vi "MSScript_SubVI_EditorShowTo.vi"(0 "Listbox Ref":refnum<vi>, 1 "Variable In":ext[](array[numeric]), 2 "Variable Index":i32[](array[numeric]), 3 "Variable Name":string, 11 "error in (no error)":errorcluster, 12 "String Color":u32) -> (15 "error out":errorcluster)   [LabVIEW 2018, in "MSScript.lvclass"]
uses:
  MSScript.lvclass
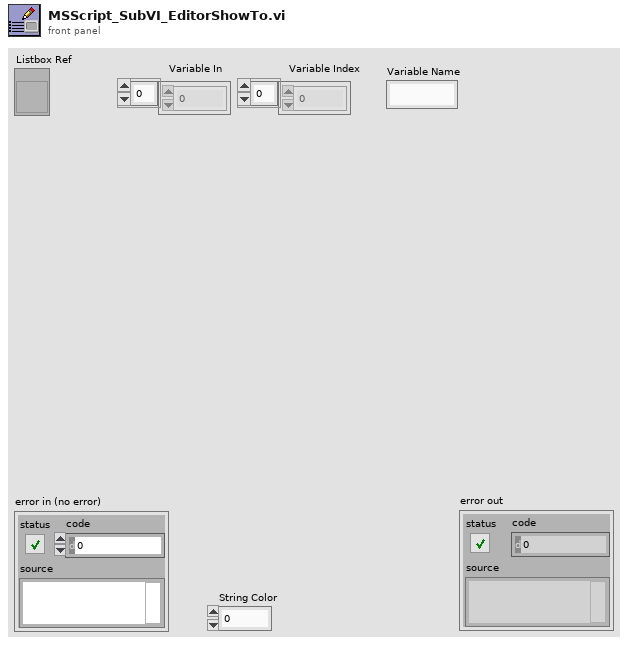
[diagram p1: front panel]
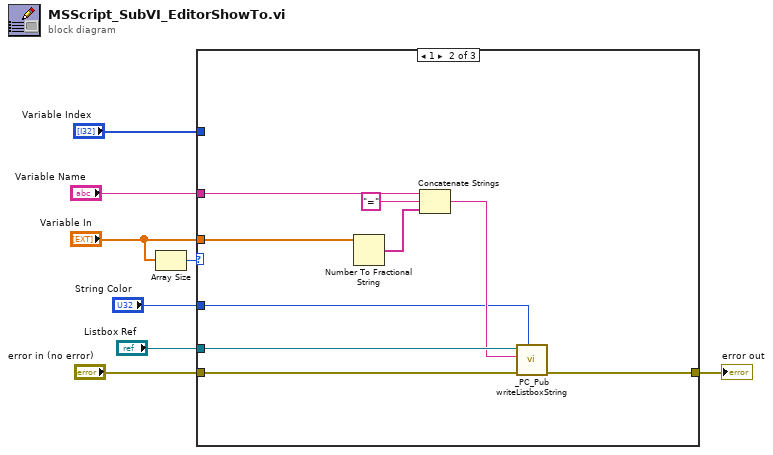
[diagram p0: block diagram]
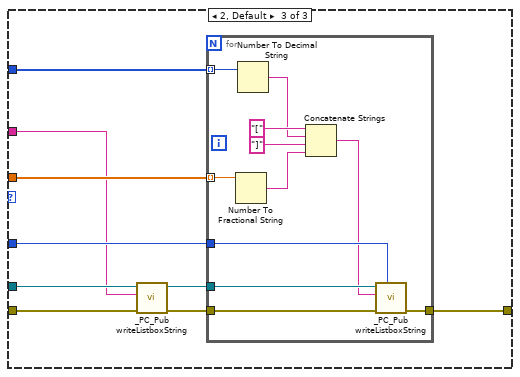
[diagram p3: hidden frame]
diagram:
  n1 = Array Size(array="Variable In") -> (size(s)=w8:i32)
  n2 = case shown="1" w8 {
    tunnel: "Variable Name" -> [_ w16 w19]
    tunnel: "Variable In" -> [_ w15 w27]
    tunnel: "Listbox Ref" -> [_ w14 w24]
    tunnel: "error in (no error)" -> [w9 w12 w23]
    tunnel: [w9 w11 w25] -> w3
    tunnel: "String Color" -> [_ w10 w26]
    tunnel: "Variable Index" -> [_ _ w20]
    frame 0 {
    }
    frame 1 {
      n3 = Number To Fractional String(number=w15) -> (F-format string=w18:string[])  [unwired: 3 in]
      n4 = Concatenate Strings(w16, "=" ("string"), w18) -> (w13:string)
      n5 = call "_PC_Pub writeListboxString.vi"("String Color"=w10, "error in (no error)"=w12, "update_Str"=w13, "Listbox Ref Input"=w14) -> ("error out"=w11:errorcluster)  [unwired: 6 in, 1 out]
    }
    frame 2, Default {
      n6 = call "_PC_Pub writeListboxString.vi"("error in (no error)"=w23, "update_Str"=w19, "Listbox Ref Input"=w24) -> ("error out"=w21:errorcluster, "Listbox Ref Output"=w22:refnum<vi>)  [unwired: 7 in]
      n7 = for {
        tunnel: w27 -> [w35] mode=indexing
        tunnel: w22 -> [w32]
        tunnel: w21 -> [w33]
        tunnel: w26 -> [w31]
        tunnel: [w30] -> w25
        tunnel: w20 -> [w28] mode=indexing
        n8 = Number To Fractional String(number=w35) -> (F-format string=w34:string)  [unwired: 3 in]
        n9 = Number To Decimal String(number=w28) -> (decimal integer string=w36:string)  [unwired: 1 in]
        n10 = Concatenate Strings("[", w36, "]", w34) -> (w29:string)
        n11 = call "_PC_Pub writeListboxString.vi"("String Color"=w31, "error in (no error)"=w33, "update_Str"=w29, "Listbox Ref Input"=w32) -> ("error out"=w30:errorcluster)  [unwired: 6 in, 1 out]
      }
    }
  }
  "error out" <- w3
